vi "TSCAN_Periodic_Sending.vi"(10 "Data":T2={"Communication message"={"Sender"="", "receiver"="", "message"="", "data"=variant}, "Data"={"Config_parameter"={"Bus_Type"=0, "Channel"=1, "Channels used"=1, "DLL_PATH"=path "", "Read message type"=1, "REC_Channel"=0}, "Send_parameter"={"SendData"=[0, 0, 0, 0, 0, 0, 0, 0, 0, 0, 0, 0, 0, 0, 0, 0, 0, 0, 0, 0, 0, 0, 0, 0, 0, 0, 0, 0, 0, 0, 0, 0, 0, 0, 0, 0, 0, 0, 0, 0, 0, 0, 0, 0, 0, 0, 0, 0, 0, 0, 0, 0, 0, 0, 0, 0, 0, 0, 0, 0, 0, 0, 0, 0, 0, 0, 0, 0, 0, 0, 0, 0, 0, 0, 0], "Data Length"=15, "ID"=0, "Frame Format"=0, "Frame Type"=0, "BRS"=enum."Close", "FD Frame"=0, "async&sync"=enum."async", "Timeout"=0}, "DBC_Ctr"={"DBC Path"=path "", "DBC loading channel"=0, "DatabaseId"=0, "DBMessages"=[], "DBSignals"=[]}, "CAN_Config_Array"=[], "CANFD_Config_Array"=[], "CAN_Config_Regs_Array"=[], "CANFD_Config_Regs_Array"=[], "Blf_Log"={"Blf_Log_PATH"=path ""}, "UDS"={"UDS Control"={"UDS Channel Index"=0, "Request ID"=1992, "Response ID"=2015, "Request ID (Func)"=1, "Session Mode"=1, "Reset Mode"=255, "DTC Mask"=0, "GropOfDTC"=0, "Seed Level"=2, "Seed"=[], "Key Level"=0, "Key"=[], "Read Identifier"=0, "UDS Read Data"=[], "ASCII Data"="", "Write Identifier"=0, "UDS Wrtie Data"=[], "IO Control Identifier"=1, "UDS IOControl Data"=[], "IO Control Mode"=0, "UDS IOControl Read Data"=[], "Routine Control Identifier"=0, "UDS RoutineControl Data"=[], "UDS RoutineControl Read Data"=[], "Routine Control Mode"=1, "SupportFDCAN"=TRUE, "time config"={"p2_timeout"=0, "p2_extended"=0, "s3_servertime"=0, "s3_clienttime"=0}, "ServiceLayer"={"FilledByte"=0, "STMin"=10, "BlockSize"=10, "FCDelay"=10, "MaxLength"=4095}, "Request"=[], "Respond"=[]}, "DiagModuleIndex"=1984}}, "CAN_Buffer"=[], "CANFD_Buffer"=[], "error in"={"status"=FALSE, "code"=0, "source"=""}, "CAN_Period_Datas"=[], "CANFD_period_Datas"=[], "CAN_Filtering_Datas"=[], "CANFD_Filtering_Datas"=[], "AsynCall?"=FALSE} {"Data"."UDS"."UDS Control"."Respond" format="%.0x"; "Data"."UDS"."UDS Control"."Request" format="%.0x"; "Data"."UDS"."UDS Control"."ServiceLayer"."FilledByte" format="%.0x"; "Data"."UDS"."UDS Control"."GropOfDTC" format="%.0x"; "Data"."UDS"."UDS Control"."DTC Mask" format="%.0x"; "Data"."UDS"."UDS Control"."UDS RoutineControl Read Data" format="%.0x"; "Data"."UDS"."UDS Control"."UDS RoutineControl Data" format="%.0x"; "Data"."UDS"."UDS Control"."Routine Control Identifier" format="%.0x"; "Data"."UDS"."UDS Control"."UDS IOControl Read Data" format="%.0x"; "Data"."UDS"."UDS Control"."UDS IOControl Data" format="%.0x"; "Data"."UDS"."UDS Control"."IO Control Identifier" format="%.0x"; "Data"."UDS"."UDS Control"."UDS Wrtie Data" format="%.0x"; "Data"."UDS"."UDS Control"."UDS Read Data" format="%.0x"; "Data"."UDS"."UDS Control"."Write Identifier" format="%.0x"; "Data"."UDS"."UDS Control"."Read Identifier" format="%.0x"; "Data"."UDS"."UDS Control"."Key" format="%.0x"; "Data"."UDS"."UDS Control"."Seed" format="%.0x"; "Data"."UDS"."UDS Control"."Request ID (Func)" format="%.0x"; "Data"."UDS"."UDS Control"."Response ID" format="%.0x"; "Data"."UDS"."UDS Control"."Request ID" format="%.0x"; "Data"."UDS"."UDS Control"."Session Mode" items=["DefaultSession"=1, "ProgrammingSession"=2, "ExtendedDiagnosticSession"=3]; "Data"."UDS"."UDS Control"."Reset Mode" items=["HardReset"=1, "keyOffOnReset"=2, "SoftReset"=3]; "Data"."UDS"."UDS Control"."IO Control Mode" items=["ReturnControlToECU", "ResetToDefault", "FreezeCurrentState", "ShortTermAdjustment"]; "Data"."UDS"."UDS Control"."Routine Control Mode" items=["Start routine"=1, "Stop routine"=2, "Request routine results"=3]; "Data"."CAN_Config_Regs_Array"."CAN configuration"."AAppChannel" items=["CHN1", "CHN2", "CHN3", "CHN4", "CHN5", "CHN6", "CHN7", "CHN8", "CHN9", "CHN10", "CHN11", "CHN12", "CHN13", "CHN14", "CHN15", "CHN16", "CHN17", "CHN18", "CHN19", "CHN20", "CHN21", "CHN22", "CHN23", "CHN24", "CHN25", "CHN26", "CHN27", "CHN28", "CHN29", "CHN30", "CHN31", "CHN32"]; "Data"."CAN_Config_Regs_Array"."CAN configuration"."AHwChannel" items=["CHN1", "CHN2", "CHN3", "CHN4", "CHN5", "CHN6", "CHN7", "CHN8", "CHN9", "CHN10", "CHN11", "CHN12", "CHN13", "CHN14", "CHN15", "CHN16", "CHN17", "CHN18", "CHN19", "CHN20", "CHN21", "CHN22", "CHN23", "CHN24", "CHN25", "CHN26", "CHN27", "CHN28", "CHN29", "CHN30", "CHN31", "CHN32"]; "Data"."CAN_Config_Regs_Array"."CAN configuration"."HardwareType" items=["BUS_UNKNOWN_TYPE", "TS_TCP_DEVICE", "XL_USB_DEVICE", "TS_USB_DEVICE", "PEAK_USB_DEVICE", "KVASER_USB_DEVICE", "ZLG_USB_DEVICE", "ICS_USB_DEVICE", "TS_TC1005_DEVICE", "CANABLE_USB_DEVICE", "TS_WIRELESS_OBD", "TS_USB_DEVICE_EX", "IXXAT_USB_DEVICE", "TS_ETH_IF_DEVICE", "TS_USB_IF_DEVICE", "BUS_DEV_TYPE_COUNT"]; "Data"."CANFD_Config_Regs_Array"."CANFD Configuration"."Hardware Type" items=["BUS_UNKNOWN_TYPE", "TS_TCP_DEVICE", "XL_USB_DEVICE", "TS_USB_DEVICE", "PEAK_USB_DEVICE", "KVASER_USB_DEVICE", "ZLG_USB_DEVICE", "ICS_USB_DEVICE", "TS_TC1005_DEVICE", "CANABLE_USB_DEVICE", "TS_WIRELESS_OBD", "TS_USB_DEVICE_EX", "IXXAT_USB_DEVICE", "TS_ETH_IF_DEVICE", "TS_USB_IF_DEVICE", "BUS_DEV_TYPE_COUNT"]; "Data"."CANFD_Config_Regs_Array"."CANFD Configuration"."AHwChannel" items=["CHN1", "CHN2", "CHN3", "CHN4", "CHN5", "CHN6", "CHN7", "CHN8", "CHN9", "CHN10", "CHN11", "CHN12", "CHN13", "CHN14", "CHN15", "CHN16", "CHN17", "CHN18", "CHN19", "CHN20", "CHN21", "CHN22", "CHN23", "CHN24", "CHN25", "CHN26", "CHN27", "CHN28", "CHN29", "CHN30", "CHN31", "CHN32"]; "Data"."CANFD_Config_Regs_Array"."CANFD Configuration"."AAppChannel" items=["CHN1", "CHN2", "CHN3", "CHN4", "CHN5", "CHN6", "CHN7", "CHN8", "CHN9", "CHN10", "CHN11", "CHN12", "CHN13", "CHN14", "CHN15", "CHN16", "CHN17", "CHN18", "CHN19", "CHN20", "CHN21", "CHN22", "CHN23", "CHN24", "CHN25", "CHN26", "CHN27", "CHN28", "CHN29", "CHN30", "CHN31", "CHN32"]; "Data"."CANFD_Config_Regs_Array"."CANFD Configuration"."AControllerType" items=["lfdtCAN", "lfdtISOFDCAN", "lfdtNonISOFDFDCAN"]; "Data"."CANFD_Config_Regs_Array"."CANFD Configuration"."AControllerMode" items=["lfdmNormal", "lfdmACKOff", "lfdmRestricted"]; "Data"."CANFD_Config_Array"."Hardware Type" items=["BUS_UNKNOWN_TYPE", "TS_TCP_DEVICE", "XL_USB_DEVICE", "TS_USB_DEVICE", "PEAK_USB_DEVICE", "KVASER_USB_DEVICE", "ZLG_USB_DEVICE", "ICS_USB_DEVICE", "TS_TC1005_DEVICE", "CANABLE_USB_DEVICE", "TS_WIRELESS_OBD", "TS_USB_DEVICE_EX", "IXXAT_USB_DEVICE", "TS_ETH_IF_DEVICE", "TS_USB_IF_DEVICE", "BUS_DEV_TYPE_COUNT"]; "Data"."CANFD_Config_Array"."AHwChannel" items=["CHN1", "CHN2", "CHN3", "CHN4", "CHN5", "CHN6", "CHN7", "CHN8", "CHN9", "CHN10", "CHN11", "CHN12", "CHN13", "CHN14", "CHN15", "CHN16", "CHN17", "CHN18", "CHN19", "CHN20", "CHN21", "CHN22", "CHN23", "CHN24", "CHN25", "CHN26", "CHN27", "CHN28", "CHN29", "CHN30", "CHN31", "CHN32"]; "Data"."CANFD_Config_Array"."AAppChannel" items=["CHN1", "CHN2", "CHN3", "CHN4", "CHN5", "CHN6", "CHN7", "CHN8", "CHN9", "CHN10", "CHN11", "CHN12", "CHN13", "CHN14", "CHN15", "CHN16", "CHN17", "CHN18", "CHN19", "CHN20", "CHN21", "CHN22", "CHN23", "CHN24", "CHN25", "CHN26", "CHN27", "CHN28", "CHN29", "CHN30", "CHN31", "CHN32"]; "Data"."CANFD_Config_Array"."AControllerType" items=["lfdtCAN", "lfdtISOFDCAN", "lfdtNonISOFDFDCAN"]; "Data"."CANFD_Config_Array"."AControllerMode" items=["lfdmNormal", "lfdmACKOff", "lfdmRestricted"]; "Data"."CAN_Config_Array"."AAppChannel" items=["CHN1", "CHN2", "CHN3", "CHN4", "CHN5", "CHN6", "CHN7", "CHN8", "CHN9", "CHN10", "CHN11", "CHN12", "CHN13", "CHN14", "CHN15", "CHN16", "CHN17", "CHN18", "CHN19", "CHN20", "CHN21", "CHN22", "CHN23", "CHN24", "CHN25", "CHN26", "CHN27", "CHN28", "CHN29", "CHN30", "CHN31", "CHN32"]; "Data"."CAN_Config_Array"."AHwChannel" items=["CHN1", "CHN2", "CHN3", "CHN4", "CHN5", "CHN6", "CHN7", "CHN8", "CHN9", "CHN10", "CHN11", "CHN12", "CHN13", "CHN14", "CHN15", "CHN16", "CHN17", "CHN18", "CHN19", "CHN20", "CHN21", "CHN22", "CHN23", "CHN24", "CHN25", "CHN26", "CHN27", "CHN28", "CHN29", "CHN30", "CHN31", "CHN32"]; "Data"."CAN_Config_Array"."HardwareType" items=["BUS_UNKNOWN_TYPE", "TS_TCP_DEVICE", "XL_USB_DEVICE", "TS_USB_DEVICE", "PEAK_USB_DEVICE", "KVASER_USB_DEVICE", "ZLG_USB_DEVICE", "ICS_USB_DEVICE", "TS_TC1005_DEVICE", "CANABLE_USB_DEVICE", "TS_WIRELESS_OBD", "TS_USB_DEVICE_EX", "IXXAT_USB_DEVICE", "TS_ETH_IF_DEVICE", "TS_USB_IF_DEVICE", "BUS_DEV_TYPE_COUNT"]; "Data"."DBC_Ctr"."DBSignals"."SignalList"."Message_Type" items=["CAN", "CANFD", "J1939"]; "Data"."DBC_Ctr"."DBSignals"."SignalList"."Mux_Type" items=["Normal", "multiplexor", "multiplexed"]; "Data"."DBC_Ctr"."DBSignals"."SignalList"."Is_Motorola" items=["Intel", "Motorola"]; "Data"."DBC_Ctr"."DBSignals"."SignalList"."Value_Type" items=["unsigned int", "signed int", "float", "double"]; "Data"."DBC_Ctr"."DBSignals"."SignalList"."ID" format="%.0x"; "Data"."DBC_Ctr"."DBMessages"."BRS" items=["No BRS", "BRS"]; "Data"."DBC_Ctr"."DBMessages"."ID" format="%.0x"; "Data"."DBC_Ctr"."DBMessages"."Type" items=["cftStdCAN", "cftExtCAN", "cftJ1939", "cftStdCANFD", "cftExtCANFD"]; "Data"."DBC_Ctr"."DBC loading channel" items=["CHN1", "CHN2", "CHN3", "CHN4", "CHN5", "CHN6", "CHN7", "CHN8", "CHN9", "CHN10", "CHN11", "CHN12", "CHN13", "CHN14", "CHN15", "CHN16", "CHN17", "CHN18", "CHN19", "CHN20", "CHN21", "CHN22", "CHN23", "CHN24", "CHN25", "CHN26", "CHN27", "CHN28", "CHN29", "CHN30", "CHN31", "CHN32"]; "Data"."Send_parameter"."FD Frame" items=["Ordinary CAN Data", "FD CAN Data"]; "Data"."Send_parameter"."Frame Type" items=["Standard Frame", "Extended Frame"]; "Data"."Send_parameter"."Frame Format" items=["Standard Frame", "Extended Frame"]; "Data"."Send_parameter"."ID" format="%x"; "Data"."Send_parameter"."Data Length" items=["0", "1", "2", "3", "4", "5", "6", "7", "8", "12", "16", "20", "24", "32", "48", "64"]; "Data"."Send_parameter"."SendData" format="%x"; "Data"."Config_parameter"."REC_Channel" items=["CHN1", "CHN2", "CHN3", "CHN4", "CHN5", "CHN6", "CHN7", "CHN8", "CHN9", "CHN10", "CHN11", "CHN12", "CHN13", "CHN14", "CHN15", "CHN16", "CHN17", "CHN18", "CHN19", "CHN20", "CHN21", "CHN22", "CHN23", "CHN24", "CHN25", "CHN26", "CHN27", "CHN28", "CHN29", "CHN30", "CHN31", "CHN32"]; "Data"."Config_parameter"."Read message type" items=["Only read received messages", "Receive&send messages"]; "Data"."Config_parameter"."Channels used" items=["1 Channel"=1, "2 Channels"=2, "3 Channels"=3, "4 Channels"=4, "5 Channels"=5, "6 Channels"=6, "7 Channels"=7, "8 Channels"=8, "9 Channels"=9, "10 Channels"=10, "11 Channels"=11, "12 Channels"=12, "13 Channels"=13, "14 Channels"=14, "15 Channels"=15, "16 Channels"=16]; "Data"."Config_parameter"."Channel" items=["Disable", "Enable"]; "Data"."Config_parameter"."Bus_Type" items=["CAN", "CANFD"]}, 11 "Sender":string="Demo") -> (2 "Data 2":T2={"Communication message"={"Sender"="", "receiver"="", "message"="", "data"=variant}, "Data"={"Config_parameter"={"Bus_Type"=0, "Channel"=1, "Channels used"=1, "DLL_PATH"=path "", "Read message type"=1, "REC_Channel"=0}, "Send_parameter"={"SendData"=[0, 0, 0, 0, 0, 0, 0, 0, 0, 0, 0, 0, 0, 0, 0, 0, 0, 0, 0, 0, 0, 0, 0, 0, 0, 0, 0, 0, 0, 0, 0, 0, 0, 0, 0, 0, 0, 0, 0, 0, 0, 0, 0, 0, 0, 0, 0, 0, 0, 0, 0, 0, 0, 0, 0, 0, 0, 0, 0, 0, 0, 0, 0, 0, 0, 0, 0, 0, 0, 0, 0, 0, 0, 0, 0], "Data Length"=15, "ID"=0, "Frame Format"=0, "Frame Type"=0, "BRS"=enum."Close", "FD Frame"=0, "async&sync"=enum."async", "Timeout"=0}, "DBC_Ctr"={"DBC Path"=path "", "DBC loading channel"=0, "DatabaseId"=0, "DBMessages"=[], "DBSignals"=[]}, "CAN_Config_Array"=[], "CANFD_Config_Array"=[], "CAN_Config_Regs_Array"=[], "CANFD_Config_Regs_Array"=[], "Blf_Log"={"Blf_Log_PATH"=path ""}, "UDS"={"UDS Control"={"UDS Channel Index"=0, "Request ID"=1992, "Response ID"=2015, "Request ID (Func)"=1, "Session Mode"=1, "Reset Mode"=255, "DTC Mask"=0, "GropOfDTC"=0, "Seed Level"=2, "Seed"=[], "Key Level"=0, "Key"=[], "Read Identifier"=0, "UDS Read Data"=[], "ASCII Data"="", "Write Identifier"=0, "UDS Wrtie Data"=[], "IO Control Identifier"=1, "UDS IOControl Data"=[], "IO Control Mode"=0, "UDS IOControl Read Data"=[], "Routine Control Identifier"=0, "UDS RoutineControl Data"=[], "UDS RoutineControl Read Data"=[], "Routine Control Mode"=1, "SupportFDCAN"=TRUE, "time config"={"p2_timeout"=0, "p2_extended"=0, "s3_servertime"=0, "s3_clienttime"=0}, "ServiceLayer"={"FilledByte"=0, "STMin"=10, "BlockSize"=10, "FCDelay"=10, "MaxLength"=4095}, "Request"=[], "Respond"=[]}, "DiagModuleIndex"=1984}}, "CAN_Buffer"=[], "CANFD_Buffer"=[], "error in"={"status"=FALSE, "code"=0, "source"=""}, "CAN_Period_Datas"=[], "CANFD_period_Datas"=[], "CAN_Filtering_Datas"=[], "CANFD_Filtering_Datas"=[], "AsynCall?"=FALSE} {"Data"."UDS"."UDS Control"."Respond" format="%.0x"; "Data"."UDS"."UDS Control"."Request" format="%.0x"; "Data"."UDS"."UDS Control"."ServiceLayer"."FilledByte" format="%.0x"; "Data"."UDS"."UDS Control"."GropOfDTC" format="%.0x"; "Data"."UDS"."UDS Control"."DTC Mask" format="%.0x"; "Data"."UDS"."UDS Control"."UDS RoutineControl Read Data" format="%.0x"; "Data"."UDS"."UDS Control"."UDS RoutineControl Data" format="%.0x"; "Data"."UDS"."UDS Control"."Routine Control Identifier" format="%.0x"; "Data"."UDS"."UDS Control"."UDS IOControl Read Data" format="%.0x"; "Data"."UDS"."UDS Control"."UDS IOControl Data" format="%.0x"; "Data"."UDS"."UDS Control"."IO Control Identifier" format="%.0x"; "Data"."UDS"."UDS Control"."UDS Wrtie Data" format="%.0x"; "Data"."UDS"."UDS Control"."UDS Read Data" format="%.0x"; "Data"."UDS"."UDS Control"."Write Identifier" format="%.0x"; "Data"."UDS"."UDS Control"."Read Identifier" format="%.0x"; "Data"."UDS"."UDS Control"."Key" format="%.0x"; "Data"."UDS"."UDS Control"."Seed" format="%.0x"; "Data"."UDS"."UDS Control"."Request ID (Func)" format="%.0x"; "Data"."UDS"."UDS Control"."Response ID" format="%.0x"; "Data"."UDS"."UDS Control"."Request ID" format="%.0x"; "Data"."UDS"."UDS Control"."Session Mode" items=["DefaultSession"=1, "ProgrammingSession"=2, "ExtendedDiagnosticSession"=3]; "Data"."UDS"."UDS Control"."Reset Mode" items=["HardReset"=1, "keyOffOnReset"=2, "SoftReset"=3]; "Data"."UDS"."UDS Control"."IO Control Mode" items=["ReturnControlToECU", "ResetToDefault", "FreezeCurrentState", "ShortTermAdjustment"]; "Data"."UDS"."UDS Control"."Routine Control Mode" items=["Start routine"=1, "Stop routine"=2, "Request routine results"=3]; "Data"."CAN_Config_Regs_Array"."CAN configuration"."AAppChannel" items=["CHN1", "CHN2", "CHN3", "CHN4", "CHN5", "CHN6", "CHN7", "CHN8", "CHN9", "CHN10", "CHN11", "CHN12", "CHN13", "CHN14", "CHN15", "CHN16", "CHN17", "CHN18", "CHN19", "CHN20", "CHN21", "CHN22", "CHN23", "CHN24", "CHN25", "CHN26", "CHN27", "CHN28", "CHN29", "CHN30", "CHN31", "CHN32"]; "Data"."CAN_Config_Regs_Array"."CAN configuration"."AHwChannel" items=["CHN1", "CHN2", "CHN3", "CHN4", "CHN5", "CHN6", "CHN7", "CHN8", "CHN9", "CHN10", "CHN11", "CHN12", "CHN13", "CHN14", "CHN15", "CHN16", "CHN17", "CHN18", "CHN19", "CHN20", "CHN21", "CHN22", "CHN23", "CHN24", "CHN25", "CHN26", "CHN27", "CHN28", "CHN29", "CHN30", "CHN31", "CHN32"]; "Data"."CAN_Config_Regs_Array"."CAN configuration"."HardwareType" items=["BUS_UNKNOWN_TYPE", "TS_TCP_DEVICE", "XL_USB_DEVICE", "TS_USB_DEVICE", "PEAK_USB_DEVICE", "KVASER_USB_DEVICE", "ZLG_USB_DEVICE", "ICS_USB_DEVICE", "TS_TC1005_DEVICE", "CANABLE_USB_DEVICE", "TS_WIRELESS_OBD", "TS_USB_DEVICE_EX", "IXXAT_USB_DEVICE", "TS_ETH_IF_DEVICE", "TS_USB_IF_DEVICE", "BUS_DEV_TYPE_COUNT"]; "Data"."CANFD_Config_Regs_Array"."CANFD Configuration"."Hardware Type" items=["BUS_UNKNOWN_TYPE", "TS_TCP_DEVICE", "XL_USB_DEVICE", "TS_USB_DEVICE", "PEAK_USB_DEVICE", "KVASER_USB_DEVICE", "ZLG_USB_DEVICE", "ICS_USB_DEVICE", "TS_TC1005_DEVICE", "CANABLE_USB_DEVICE", "TS_WIRELESS_OBD", "TS_USB_DEVICE_EX", "IXXAT_USB_DEVICE", "TS_ETH_IF_DEVICE", "TS_USB_IF_DEVICE", "BUS_DEV_TYPE_COUNT"]; "Data"."CANFD_Config_Regs_Array"."CANFD Configuration"."AHwChannel" items=["CHN1", "CHN2", "CHN3", "CHN4", "CHN5", "CHN6", "CHN7", "CHN8", "CHN9", "CHN10", "CHN11", "CHN12", "CHN13", "CHN14", "CHN15", "CHN16", "CHN17", "CHN18", "CHN19", "CHN20", "CHN21", "CHN22", "CHN23", "CHN24", "CHN25", "CHN26", "CHN27", "CHN28", "CHN29", "CHN30", "CHN31", "CHN32"]; "Data"."CANFD_Config_Regs_Array"."CANFD Configuration"."AAppChannel" items=["CHN1", "CHN2", "CHN3", "CHN4", "CHN5", "CHN6", "CHN7", "CHN8", "CHN9", "CHN10", "CHN11", "CHN12", "CHN13", "CHN14", "CHN15", "CHN16", "CHN17", "CHN18", "CHN19", "CHN20", "CHN21", "CHN22", "CHN23", "CHN24", "CHN25", "CHN26", "CHN27", "CHN28", "CHN29", "CHN30", "CHN31", "CHN32"]; "Data"."CANFD_Config_Regs_Array"."CANFD Configuration"."AControllerType" items=["lfdtCAN", "lfdtISOFDCAN", "lfdtNonISOFDFDCAN"]; "Data"."CANFD_Config_Regs_Array"."CANFD Configuration"."AControllerMode" items=["lfdmNormal", "lfdmACKOff", "lfdmRestricted"]; "Data"."CANFD_Config_Array"."Hardware Type" items=["BUS_UNKNOWN_TYPE", "TS_TCP_DEVICE", "XL_USB_DEVICE", "TS_USB_DEVICE", "PEAK_USB_DEVICE", "KVASER_USB_DEVICE", "ZLG_USB_DEVICE", "ICS_USB_DEVICE", "TS_TC1005_DEVICE", "CANABLE_USB_DEVICE", "TS_WIRELESS_OBD", "TS_USB_DEVICE_EX", "IXXAT_USB_DEVICE", "TS_ETH_IF_DEVICE", "TS_USB_IF_DEVICE", "BUS_DEV_TYPE_COUNT"]; "Data"."CANFD_Config_Array"."AHwChannel" items=["CHN1", "CHN2", "CHN3", "CHN4", "CHN5", "CHN6", "CHN7", "CHN8", "CHN9", "CHN10", "CHN11", "CHN12", "CHN13", "CHN14", "CHN15", "CHN16", "CHN17", "CHN18", "CHN19", "CHN20", "CHN21", "CHN22", "CHN23", "CHN24", "CHN25", "CHN26", "CHN27", "CHN28", "CHN29", "CHN30", "CHN31", "CHN32"]; "Data"."CANFD_Config_Array"."AAppChannel" items=["CHN1", "CHN2", "CHN3", "CHN4", "CHN5", "CHN6", "CHN7", "CHN8", "CHN9", "CHN10", "CHN11", "CHN12", "CHN13", "CHN14", "CHN15", "CHN16", "CHN17", "CHN18", "CHN19", "CHN20", "CHN21", "CHN22", "CHN23", "CHN24", "CHN25", "CHN26", "CHN27", "CHN28", "CHN29", "CHN30", "CHN31", "CHN32"]; "Data"."CANFD_Config_Array"."AControllerType" items=["lfdtCAN", "lfdtISOFDCAN", "lfdtNonISOFDFDCAN"]; "Data"."CANFD_Config_Array"."AControllerMode" items=["lfdmNormal", "lfdmACKOff", "lfdmRestricted"]; "Data"."CAN_Config_Array"."AAppChannel" items=["CHN1", "CHN2", "CHN3", "CHN4", "CHN5", "CHN6", "CHN7", "CHN8", "CHN9", "CHN10", "CHN11", "CHN12", "CHN13", "CHN14", "CHN15", "CHN16", "CHN17", "CHN18", "CHN19", "CHN20", "CHN21", "CHN22", "CHN23", "CHN24", "CHN25", "CHN26", "CHN27", "CHN28", "CHN29", "CHN30", "CHN31", "CHN32"]; "Data"."CAN_Config_Array"."AHwChannel" items=["CHN1", "CHN2", "CHN3", "CHN4", "CHN5", "CHN6", "CHN7", "CHN8", "CHN9", "CHN10", "CHN11", "CHN12", "CHN13", "CHN14", "CHN15", "CHN16", "CHN17", "CHN18", "CHN19", "CHN20", "CHN21", "CHN22", "CHN23", "CHN24", "CHN25", "CHN26", "CHN27", "CHN28", "CHN29", "CHN30", "CHN31", "CHN32"]; "Data"."CAN_Config_Array"."HardwareType" items=["BUS_UNKNOWN_TYPE", "TS_TCP_DEVICE", "XL_USB_DEVICE", "TS_USB_DEVICE", "PEAK_USB_DEVICE", "KVASER_USB_DEVICE", "ZLG_USB_DEVICE", "ICS_USB_DEVICE", "TS_TC1005_DEVICE", "CANABLE_USB_DEVICE", "TS_WIRELESS_OBD", "TS_USB_DEVICE_EX", "IXXAT_USB_DEVICE", "TS_ETH_IF_DEVICE", "TS_USB_IF_DEVICE", "BUS_DEV_TYPE_COUNT"]; "Data"."DBC_Ctr"."DBSignals"."SignalList"."Message_Type" items=["CAN", "CANFD", "J1939"]; "Data"."DBC_Ctr"."DBSignals"."SignalList"."Mux_Type" items=["Normal", "multiplexor", "multiplexed"]; "Data"."DBC_Ctr"."DBSignals"."SignalList"."Is_Motorola" items=["Intel", "Motorola"]; "Data"."DBC_Ctr"."DBSignals"."SignalList"."Value_Type" items=["unsigned int", "signed int", "float", "double"]; "Data"."DBC_Ctr"."DBSignals"."SignalList"."ID" format="%.0x"; "Data"."DBC_Ctr"."DBMessages"."BRS" items=["No BRS", "BRS"]; "Data"."DBC_Ctr"."DBMessages"."ID" format="%.0x"; "Data"."DBC_Ctr"."DBMessages"."Type" items=["cftStdCAN", "cftExtCAN", "cftJ1939", "cftStdCANFD", "cftExtCANFD"]; "Data"."DBC_Ctr"."DBC loading channel" items=["CHN1", "CHN2", "CHN3", "CHN4", "CHN5", "CHN6", "CHN7", "CHN8", "CHN9", "CHN10", "CHN11", "CHN12", "CHN13", "CHN14", "CHN15", "CHN16", "CHN17", "CHN18", "CHN19", "CHN20", "CHN21", "CHN22", "CHN23", "CHN24", "CHN25", "CHN26", "CHN27", "CHN28", "CHN29", "CHN30", "CHN31", "CHN32"]; "Data"."Send_parameter"."FD Frame" items=["Ordinary CAN Data", "FD CAN Data"]; "Data"."Send_parameter"."Frame Type" items=["Standard Frame", "Extended Frame"]; "Data"."Send_parameter"."Frame Format" items=["Standard Frame", "Extended Frame"]; "Data"."Send_parameter"."ID" format="%x"; "Data"."Send_parameter"."Data Length" items=["0", "1", "2", "3", "4", "5", "6", "7", "8", "12", "16", "20", "24", "32", "48", "64"]; "Data"."Send_parameter"."SendData" format="%x"; "Data"."Config_parameter"."REC_Channel" items=["CHN1", "CHN2", "CHN3", "CHN4", "CHN5", "CHN6", "CHN7", "CHN8", "CHN9", "CHN10", "CHN11", "CHN12", "CHN13", "CHN14", "CHN15", "CHN16", "CHN17", "CHN18", "CHN19", "CHN20", "CHN21", "CHN22", "CHN23", "CHN24", "CHN25", "CHN26", "CHN27", "CHN28", "CHN29", "CHN30", "CHN31", "CHN32"]; "Data"."Config_parameter"."Read message type" items=["Only read received messages", "Receive&send messages"]; "Data"."Config_parameter"."Channels used" items=["1 Channel"=1, "2 Channels"=2, "3 Channels"=3, "4 Channels"=4, "5 Channels"=5, "6 Channels"=6, "7 Channels"=7, "8 Channels"=8, "9 Channels"=9, "10 Channels"=10, "11 Channels"=11, "12 Channels"=12, "13 Channels"=13, "14 Channels"=14, "15 Channels"=15, "16 Channels"=16]; "Data"."Config_parameter"."Channel" items=["Disable", "Enable"]; "Data"."Config_parameter"."Bus_Type" items=["CAN", "CANFD"]})   [LabVIEW 2014]
uses:
  <vilib>/Utility/miscctls.llb/LVPointTypeDef.ctl
  Typedef/TSCAN_Config_parameter.ctl
  Typedef/TSCAN_Send_parameter.ctl
  Typedef/TSCAN_DBC_Ctr.ctl
  Utilities/Typedef/Hardware_Subtype.ctl
  Typedef/TSCAN_CAN_Configuration.ctl
  Typedef/TSCAN_CANFD_Configuration.ctl
  Typedef/TSCAN_CAN_CANFD_Demo_Data.ctl
  Typedef/TSCAN_CAN_CANFD_Demo_Data1.ctl
  Typedef/TLibCANFD.ctl
  Typedef/TLibCAN.ctl
  Typedef/TSCAN_CANFD_Configuration_Regs.ctl
  Typedef/TSCAN_CAN_Configuration_Regs.ctl
  All_Control/Typedef/Hardware Type.ctl
  All_Control/Typedef/Blf_Log.ctl
  DataBase/Typedef/DBSignal.ctl
  DataBase/Typedef/DBMessage.ctl
  Diagnosis/Typedef/UDS Control.ctl
  Diagnosis/Typedef/UDS Cluster.ctl
panel:
  in  "Channel":i32(ring) items=["CHN1", "CHN2", "CHN3", "CHN4", "CHN5", "CHN6", "CHN7", "CHN8", "CHN9", "CHN10", "CHN11", "CHN12", "CHN13", "CHN14", "CHN15", "CHN16", "CHN17", "CHN18", "CHN19", "CHN20", "CHN21", "CHN22", "CHN23", "CHN24", "CHN25", "CHN26", "CHN27", "CHN28", "CHN29", "CHN30", "CHN31", "CHN32"]
  out "CAN_Period_Datas":T1(array[cluster])
  in  "APeriodMS":dbl
  in  "BRS":enum16{"Close", "Open"}(ring)
  in  "FD Frame":u8(ring) items=["Ordinary CAN Data", "FD CAN Data"]
  in  "Frame Type":u8(ring) items=["Data Frame", "Remote Frame", ""]
  in  "Frame Format":u8(ring) items=["Standard Frame", "Extended Frame"]
  in  "ID":i32 format="%x"
  in  "Data Length":i32(ring)=15 items=["0", "1", "2", "3", "4", "5", "6", "7", "8", "12", "16", "20", "24", "32", "48", "64"]
  in  "SendData":u8[](array[numeric])=[0, 0, 0, 0, 0, 0, 0, 0, 0, 0, 0, 0, 0, 0, 0, 0, 0, 0, 0, 0, 0, 0, 0, 0, 0, 0, 0, 0, 0, 0, 0, 0, 0, 0, 0, 0, 0, 0, 0, 0, 0, 0, 0, 0, 0, 0, 0, 0, 0, 0, 0, 0, 0, 0, 0, 0, 0, 0, 0, 0, 0, 0, 0, 0, 0, 0, 0, 0, 0, 0, 0, 0, 0, 0, 0] format="%x"
  in  "Data_Display":i32(listbox)=-1
  in  "Remove":bool
  in  "Add":bool
  in  "STOP":bool
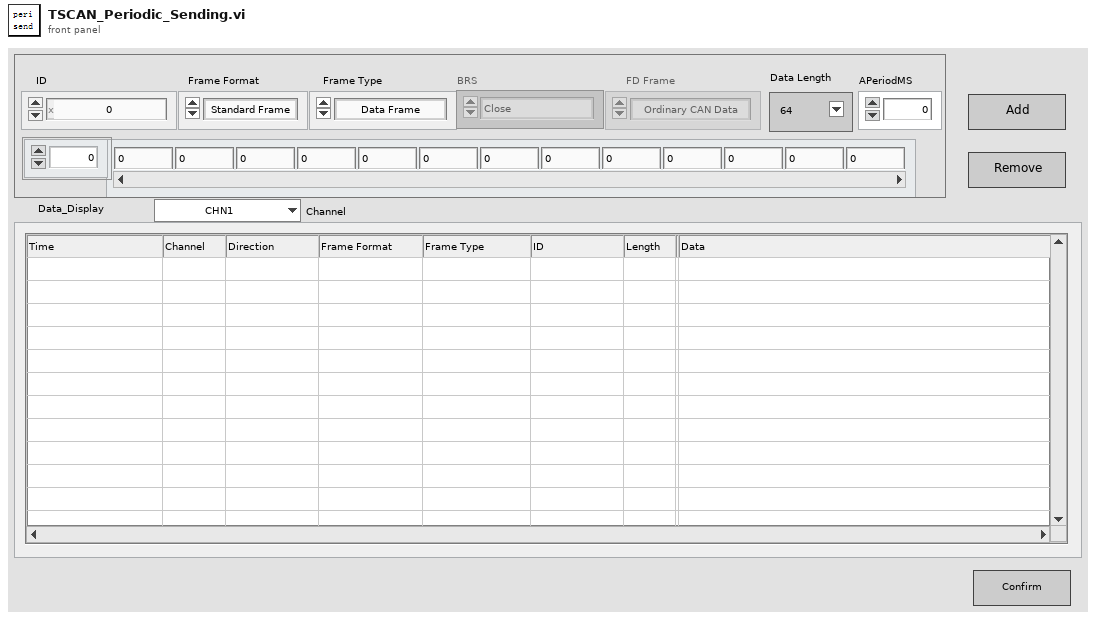
[diagram p1: front panel]
types:
  T1 = cluster{"FIdxChn":u8, "FProperties":u8, "FDLC":u8, "FReserved":u8, "FIdentifier":i32, "FTimeUS":u64, "FData":cluster{"Data0":u8, "Data1":u8, "Data2":u8, "Data3":u8, "Data4":u8, "Data5":u8, "Data6":u8, "Data7":u8}}[]
  T2 = typedef "TSCAN_CAN_CANFD_Demo_Data1.ctl" = cluster{"Communication message":cluster{"Sender":string, "receiver":string, "message":string, "data":variant}, "Data":T3, "CAN_Buffer":cluster{"FIdxChn":u8, "FProperties":u8, "FDLC":u8, "FReserved":u8, "FIdentifier":i32, "FTimeUS":u64, "FData":cluster{"Data0":u8, "Data1":u8, "Data2":u8, "Data3":u8, "Data4":u8, "Data5":u8, "Data6":u8, "Data7":u8}}[], "CANFD_Buffer":cluster{"FIdxChn":u8, "FProperties":u8, "FDLC":u8, "FReserved":u8, "FIdentifier":i32, "FTimeUS":u64, "FDatas":cluster{"Initialize array[0]":u8, "Initialize array[1]":u8, "Initialize array[2]":u8, "Initialize array[3]":u8, "Initialize array[4]":u8, "Initialize array[5]":u8, "Initialize array[6]":u8, "Initialize array[7]":u8, "Initialize array[8]":u8, "Initialize array[9]":u8, "Initialize array[10]":u8, "Initialize array[11]":u8, "Initialize array[12]":u8, "Initialize array[13]":u8, "Initialize array[14]":u8, "Initialize array[15]":u8, "Initialize array[16]":u8, "Initialize array[17]":u8, "Initialize array[18]":u8, "Initialize array[19]":u8, "Initialize array[20]":u8, "Initialize array[21]":u8, "Initialize array[22]":u8, "Initialize array[23]":u8, "Initialize array[24]":u8, "Initialize array[25]":u8, "Initialize array[26]":u8, "Initialize array[27]":u8, "Initialize array[28]":u8, "Initialize array[29]":u8, "Initialize array[30]":u8, "Initialize array[31]":u8, "Initialize array[32]":u8, "Initialize array[33]":u8, "Initialize array[34]":u8, "Initialize array[35]":u8, "Initialize array[36]":u8, "Initialize array[37]":u8, "Initialize array[38]":u8, "Initialize array[39]":u8, "Initialize array[40]":u8, "Initialize array[41]":u8, "Initialize array[42]":u8, "Initialize array[43]":u8, "Initialize array[44]":u8, "Initialize array[45]":u8, "Initialize array[46]":u8, "Initialize array[47]":u8, "Initialize array[48]":u8, "Initialize array[49]":u8, "Initialize array[50]":u8, "Initialize array[51]":u8, "Initialize array[52]":u8, "Initialize array[53]":u8, "Initialize array[54]":u8, "Initialize array[55]":u8, "Initialize array[56]":u8, "Initialize array[57]":u8, "Initialize array[58]":u8, "Initialize array[59]":u8, "Initialize array[60]":u8, "Initialize array[61]":u8, "Initialize array[62]":u8, "Initialize array[63]":u8}}[], "error in":errorcluster, "CAN_Period_Datas":cluster{"FIdxChn":u8, "FProperties":u8, "FDLC":u8, "FReserved":u8, "FIdentifier":i32, "FTimeUS":u64, "FData":cluster{"Data0":u8, "Data1":u8, "Data2":u8, "Data3":u8, "Data4":u8, "Data5":u8, "Data6":u8, "Data7":u8}}[], "CANFD_period_Datas":cluster{"FIdxChn":u8, "FProperties":u8, "FDLC":u8, "FReserved":u8, "FIdentifier":i32, "FTimeUS":u64, "FDatas":cluster{"Initialize array[0]":u8, "Initialize array[1]":u8, "Initialize array[2]":u8, "Initialize array[3]":u8, "Initialize array[4]":u8, "Initialize array[5]":u8, "Initialize array[6]":u8, "Initialize array[7]":u8, "Initialize array[8]":u8, "Initialize array[9]":u8, "Initialize array[10]":u8, "Initialize array[11]":u8, "Initialize array[12]":u8, "Initialize array[13]":u8, "Initialize array[14]":u8, "Initialize array[15]":u8, "Initialize array[16]":u8, "Initialize array[17]":u8, "Initialize array[18]":u8, "Initialize array[19]":u8, "Initialize array[20]":u8, "Initialize array[21]":u8, "Initialize array[22]":u8, "Initialize array[23]":u8, "Initialize array[24]":u8, "Initialize array[25]":u8, "Initialize array[26]":u8, "Initialize array[27]":u8, "Initialize array[28]":u8, "Initialize array[29]":u8, "Initialize array[30]":u8, "Initialize array[31]":u8, "Initialize array[32]":u8, "Initialize array[33]":u8, "Initialize array[34]":u8, "Initialize array[35]":u8, "Initialize array[36]":u8, "Initialize array[37]":u8, "Initialize array[38]":u8, "Initialize array[39]":u8, "Initialize array[40]":u8, "Initialize array[41]":u8, "Initialize array[42]":u8, "Initialize array[43]":u8, "Initialize array[44]":u8, "Initialize array[45]":u8, "Initialize array[46]":u8, "Initialize array[47]":u8, "Initialize array[48]":u8, "Initialize array[49]":u8, "Initialize array[50]":u8, "Initialize array[51]":u8, "Initialize array[52]":u8, "Initialize array[53]":u8, "Initialize array[54]":u8, "Initialize array[55]":u8, "Initialize array[56]":u8, "Initialize array[57]":u8, "Initialize array[58]":u8, "Initialize array[59]":u8, "Initialize array[60]":u8, "Initialize array[61]":u8, "Initialize array[62]":u8, "Initialize array[63]":u8}}[], "CAN_Filtering_Datas":cluster{"FIdxChn":u8, "FProperties":u8, "FDLC":u8, "FReserved":u8, "FIdentifier":i32, "FTimeUS":u64, "FData":cluster{"Data0":u8, "Data1":u8, "Data2":u8, "Data3":u8, "Data4":u8, "Data5":u8, "Data6":u8, "Data7":u8}}[], "CANFD_Filtering_Datas":cluster{"FIdxChn":u8, "FProperties":u8, "FDLC":u8, "FReserved":u8, "FIdentifier":i32, "FTimeUS":u64, "FDatas":cluster{"Initialize array[0]":u8, "Initialize array[1]":u8, "Initialize array[2]":u8, "Initialize array[3]":u8, "Initialize array[4]":u8, "Initialize array[5]":u8, "Initialize array[6]":u8, "Initialize array[7]":u8, "Initialize array[8]":u8, "Initialize array[9]":u8, "Initialize array[10]":u8, "Initialize array[11]":u8, "Initialize array[12]":u8, "Initialize array[13]":u8, "Initialize array[14]":u8, "Initialize array[15]":u8, "Initialize array[16]":u8, "Initialize array[17]":u8, "Initialize array[18]":u8, "Initialize array[19]":u8, "Initialize array[20]":u8, "Initialize array[21]":u8, "Initialize array[22]":u8, "Initialize array[23]":u8, "Initialize array[24]":u8, "Initialize array[25]":u8, "Initialize array[26]":u8, "Initialize array[27]":u8, "Initialize array[28]":u8, "Initialize array[29]":u8, "Initialize array[30]":u8, "Initialize array[31]":u8, "Initialize array[32]":u8, "Initialize array[33]":u8, "Initialize array[34]":u8, "Initialize array[35]":u8, "Initialize array[36]":u8, "Initialize array[37]":u8, "Initialize array[38]":u8, "Initialize array[39]":u8, "Initialize array[40]":u8, "Initialize array[41]":u8, "Initialize array[42]":u8, "Initialize array[43]":u8, "Initialize array[44]":u8, "Initialize array[45]":u8, "Initialize array[46]":u8, "Initialize array[47]":u8, "Initialize array[48]":u8, "Initialize array[49]":u8, "Initialize array[50]":u8, "Initialize array[51]":u8, "Initialize array[52]":u8, "Initialize array[53]":u8, "Initialize array[54]":u8, "Initialize array[55]":u8, "Initialize array[56]":u8, "Initialize array[57]":u8, "Initialize array[58]":u8, "Initialize array[59]":u8, "Initialize array[60]":u8, "Initialize array[61]":u8, "Initialize array[62]":u8, "Initialize array[63]":u8}}[], "AsynCall?":bool}
  T3 = typedef "TSCAN_CAN_CANFD_Demo_Data.ctl" = cluster{"Config_parameter":T4, "Send_parameter":T5, "DBC_Ctr":T6, "CAN_Config_Array":T9[], "CANFD_Config_Array":T12[], "CAN_Config_Regs_Array":T13[], "CANFD_Config_Regs_Array":T14[], "Blf_Log":T15, "UDS":T16}
  T4 = typedef "TSCAN_Config_parameter.ctl" = cluster{"Bus_Type":u16, "Channel":i32, "Channels used":u16, "DLL_PATH":path, "Read message type":u16, "REC_Channel":i32}
  T5 = typedef "TSCAN_Send_parameter.ctl" = cluster{"SendData":u8[], "Data Length":i32, "ID":i32, "Frame Format":u8, "Frame Type":u8, "BRS":enum16{"Close", "Open"}, "FD Frame":u8, "async&sync":enum16{"async", "sync"}, "Timeout":u16}
  T6 = typedef "TSCAN_DBC_Ctr.ctl" = cluster{"DBC Path":path, "DBC loading channel":i32, "DatabaseId":u32, "DBMessages":T7[], "DBSignals":cluster{"MessageName":string, "SignalList":T8[]}[]}
  T7 = typedef "DBMessage.ctl" = cluster{"Type":u16, "DLC":i32, "ID":i32, "CycleTime":dbl, "Name":string, "Comment":string, "TX_Node_Index":i32, "Owned_Signal_List_Count ":i32, "Owned_Signal_List_Signal_Index":i32, "BRS":i32}
  T8 = typedef "DBSignal.ctl" = cluster{"ID":i32, "Value_Type":i32, "Is_Motorola":i32, "ValTab_Index":i32, "Mux_Type":i32, "Mux_Value":dbl, "Layout_Start":i32, "Length":i32, "Factor":dbl, "Offset":dbl, "InitValue":dbl, "Min":dbl, "Max":dbl, "Name":string, "Unit":string, "Comment":string, "Message_Index":i32, "Message_Type":i32}
  T9 = typedef "TSCAN_CAN_Configuration.ctl" = cluster{"HardwareType":T10, "Hardware Subtype":T11, "ABaudrateKbps":sgl, "AListenOnly":enum16{"Normal", "ListenOnly"}, "Int120Ohm":enum16{"Disable", "Enable"}, "EnableChannel":enum16{"Disable", "Enable"}, "AHwChannel":i32, "AAppChannel":i32, "AldHW":i32}
  T10 = typedef "Hardware Type.ctl" = i32
  T11 = typedef "Hardware_Subtype.ctl" = enum16{"TS_UNKNOWN_DEVICE", "TSCAN_PRO", "TSCAN_Lite1", "TC1001", "TL1001", "TC1011", "TM5011", "TC1002", "TC1014", "TSCANFD2517", "TC1026", "TC1016", "TC1012", "TC1013", "TLog1002", "TC1034", "TC1018", "GW2116", "TC2115", "MP1013", "TC1113", "TC1114", "TP1013", "TC1017", "TP1018", "TF10XX", "TL1004_FD_4_LIN_2", "TE1051", "TP1051", "TP1034", "TTS9015", "TP1026", "TTS1026", "TTS1034", "TTS1018", "TL1011", "TTS1015_LiAuto", "TTS1013_LiAuto", "TTS1016Pro", "TC1054Pro", "TC1054", "TLog1038", "TO1013", "TC1034Pro", "TC1018Pro", "TC1038Pro", "TS_DEV_END"}
  T12 = typedef "TSCAN_CANFD_Configuration.ctl" = cluster{"Hardware Type":T10, "Hardware Subtype":T11, "AArbRateKbps":sgl, "AListenOnly":enum16{"Normal", "ListenOnly"}, "Int120Ohm":enum16{"Disable", "Enable"}, "EnableChannel":enum16{"Disable", "Enable"}, "AHwChannel":i32, "AAppChannel":i32, "ADataRateKbps":sgl, "AControllerType":i32, "AControllerMode":i32, "AldHW":i32}
  T13 = typedef "TSCAN_CAN_Configuration_Regs.ctl" = cluster{"CAN_Sampling point":cluster{"ASEG1":i32, "ASEG2":i32, "APrescaler":i32, "ASJW":i32}, "CAN configuration":T9}
  T14 = typedef "TSCAN_CANFD_Configuration_Regs.ctl" = cluster{"CANFD Configuration":T12, "CANFD_Sampling point":cluster{"AArbSEG1":i32, "AArbSEG2":i32, "AArbPrescaler":i32, "AArbSJW":i32, "ADataSEG1":i32, "ADataSEG2":i32, "ADataPrescaler":i32, "ADataSJW":i32}}
  T15 = typedef "Blf_Log.ctl" = cluster{"Blf_Log_PATH":path}
  T16 = typedef "UDS Cluster.ctl" = cluster{"UDS Control":T17, "DiagModuleIndex":i32}
  T17 = typedef "UDS Control.ctl" = cluster{"UDS Channel Index":u32, "Request ID":u32, "Response ID":u32, "Request ID (Func)":u32, "Session Mode":u8, "Reset Mode":u8, "DTC Mask":u8, "GropOfDTC":u32, "Seed Level":i32, "Seed":u8[], "Key Level":i32, "Key":u8[], "Read Identifier":u16, "UDS Read Data":u8[], "ASCII Data":string, "Write Identifier":u16, "UDS Wrtie Data":u8[], "IO Control Identifier":u16, "UDS IOControl Data":u8[], "IO Control Mode":u8, "UDS IOControl Read Data":u8[], "Routine Control Identifier":u16, "UDS RoutineControl Data":u8[], "UDS RoutineControl Read Data":u8[], "Routine Control Mode":u8, "SupportFDCAN":bool, "time config":cluster{"p2_timeout":i32, "p2_extended":i32, "s3_servertime":i32, "s3_clienttime":i32}, "ServiceLayer":cluster{"FilledByte":u8, "STMin":i32, "BlockSize":i32, "FCDelay":i32, "MaxLength":i32}, "Request":u8[], "Respond":u8[]}
  T18 = cluster{"Sender":string, "receiver":string, "message":string, "data":variant}
  T19 = typedef "LVPointTypeDef.ctl" = cluster{"Horizontal":i16, "Vertical":i16}
  T20 = enum8{"Enabled", "Disabled", "Disabled and Grayed Out"}
  T21 = cluster{"FIdxChn":u8, "FProperties":u8, "FDLC":u8, "FReserved":u8, "FIdentifier":i32, "FTimeUS":u64, "FDatas":cluster{"Initialize array[0]":u8, "Initialize array[1]":u8, "Initialize array[2]":u8, "Initialize array[3]":u8, "Initialize array[4]":u8, "Initialize array[5]":u8, "Initialize array[6]":u8, "Initialize array[7]":u8, "Initialize array[8]":u8, "Initialize array[9]":u8, "Initialize array[10]":u8, "Initialize array[11]":u8, "Initialize array[12]":u8, "Initialize array[13]":u8, "Initialize array[14]":u8, "Initialize array[15]":u8, "Initialize array[16]":u8, "Initialize array[17]":u8, "Initialize array[18]":u8, "Initialize array[19]":u8, "Initialize array[20]":u8, "Initialize array[21]":u8, "Initialize array[22]":u8, "Initialize array[23]":u8, "Initialize array[24]":u8, "Initialize array[25]":u8, "Initialize array[26]":u8, "Initialize array[27]":u8, "Initialize array[28]":u8, "Initialize array[29]":u8, "Initialize array[30]":u8, "Initialize array[31]":u8, "Initialize array[32]":u8, "Initialize array[33]":u8, "Initialize array[34]":u8, "Initialize array[35]":u8, "Initialize array[36]":u8, "Initialize array[37]":u8, "Initialize array[38]":u8, "Initialize array[39]":u8, "Initialize array[40]":u8, "Initialize array[41]":u8, "Initialize array[42]":u8, "Initialize array[43]":u8, "Initialize array[44]":u8, "Initialize array[45]":u8, "Initialize array[46]":u8, "Initialize array[47]":u8, "Initialize array[48]":u8, "Initialize array[49]":u8, "Initialize array[50]":u8, "Initialize array[51]":u8, "Initialize array[52]":u8, "Initialize array[53]":u8, "Initialize array[54]":u8, "Initialize array[55]":u8, "Initialize array[56]":u8, "Initialize array[57]":u8, "Initialize array[58]":u8, "Initialize array[59]":u8, "Initialize array[60]":u8, "Initialize array[61]":u8, "Initialize array[62]":u8, "Initialize array[63]":u8}}[]
  T22 = typedef "TLibCAN.ctl" = cluster{"AIdxchn":u8, "AId":i32, "AIsStd":u8, "AIsData":u8, "ADLC":u8, "ADataArray":cluster{"Data0":u8, "Data1":u8, "Data2":u8, "Data3":u8, "Data4":u8, "Data5":u8, "Data6":u8, "Data7":u8}}
  T23 = typedef "TLibCANFD.ctl" = cluster{"AIdxchn":u8, "AId":i32, "AIsStd":u8, "BRS":enum16{"Close", "Open"}, "AIsData":u8, "ADLC":i32, "AIsFD":enum16{"Classic CAN Message", "FD CAN Message"}, "FDatas":cluster{"Initialize array[0]":u8, "Initialize array[1]":u8, "Initialize array[2]":u8, "Initialize array[3]":u8, "Initialize array[4]":u8, "Initialize array[5]":u8, "Initialize array[6]":u8, "Initialize array[7]":u8, "Initialize array[8]":u8, "Initialize array[9]":u8, "Initialize array[10]":u8, "Initialize array[11]":u8, "Initialize array[12]":u8, "Initialize array[13]":u8, "Initialize array[14]":u8, "Initialize array[15]":u8, "Initialize array[16]":u8, "Initialize array[17]":u8, "Initialize array[18]":u8, "Initialize array[19]":u8, "Initialize array[20]":u8, "Initialize array[21]":u8, "Initialize array[22]":u8, "Initialize array[23]":u8, "Initialize array[24]":u8, "Initialize array[25]":u8, "Initialize array[26]":u8, "Initialize array[27]":u8, "Initialize array[28]":u8, "Initialize array[29]":u8, "Initialize array[30]":u8, "Initialize array[31]":u8, "Initialize array[32]":u8, "Initialize array[33]":u8, "Initialize array[34]":u8, "Initialize array[35]":u8, "Initialize array[36]":u8, "Initialize array[37]":u8, "Initialize array[38]":u8, "Initialize array[39]":u8, "Initialize array[40]":u8, "Initialize array[41]":u8, "Initialize array[42]":u8, "Initialize array[43]":u8, "Initialize array[44]":u8, "Initialize array[45]":u8, "Initialize array[46]":u8, "Initialize array[47]":u8, "Initialize array[48]":u8, "Initialize array[49]":u8, "Initialize array[50]":u8, "Initialize array[51]":u8, "Initialize array[52]":u8, "Initialize array[53]":u8, "Initialize array[54]":u8, "Initialize array[55]":u8, "Initialize array[56]":u8, "Initialize array[57]":u8, "Initialize array[58]":u8, "Initialize array[59]":u8, "Initialize array[60]":u8, "Initialize array[61]":u8, "Initialize array[62]":u8, "Initialize array[63]":u8}}
  T24 = cluster{"SendData[0]":u8, "SendData[1]":u8, "SendData[2]":u8, "SendData[3]":u8, "SendData[4]":u8, "SendData[5]":u8, "SendData[6]":u8, "SendData[7]":u8}
  T25 = cluster{"SendData[0]":u8, "SendData[1]":u8, "SendData[2]":u8, "SendData[3]":u8, "SendData[4]":u8, "SendData[5]":u8, "SendData[6]":u8, "SendData[7]":u8, "SendData[8]":u8, "SendData[9]":u8, "SendData[10]":u8, "SendData[11]":u8, "SendData[12]":u8, "SendData[13]":u8, "SendData[14]":u8, "SendData[15]":u8, "SendData[16]":u8, "SendData[17]":u8, "SendData[18]":u8, "SendData[19]":u8, "SendData[20]":u8, "SendData[21]":u8, "SendData[22]":u8, "SendData[23]":u8, "SendData[24]":u8, "SendData[25]":u8, "SendData[26]":u8, "SendData[27]":u8, "SendData[28]":u8, "SendData[29]":u8, "SendData[30]":u8, "SendData[31]":u8, "SendData[32]":u8, "SendData[33]":u8, "SendData[34]":u8, "SendData[35]":u8, "SendData[36]":u8, "SendData[37]":u8, "SendData[38]":u8, "SendData[39]":u8, "SendData[40]":u8, "SendData[41]":u8, "SendData[42]":u8, "SendData[43]":u8, "SendData[44]":u8, "SendData[45]":u8, "SendData[46]":u8, "SendData[47]":u8, "SendData[48]":u8, "SendData[49]":u8, "SendData[50]":u8, "SendData[51]":u8, "SendData[52]":u8, "SendData[53]":u8, "SendData[54]":u8, "SendData[55]":u8, "SendData[56]":u8, "SendData[57]":u8, "SendData[58]":u8, "SendData[59]":u8, "SendData[60]":u8, "SendData[61]":u8, "SendData[62]":u8, "SendData[63]":u8}
  T26 = enum32{"invalid app kind", "Development System", "Run Time System", "Student Edition", "Embedded LabVIEW", "Evaluation", "Custom"}
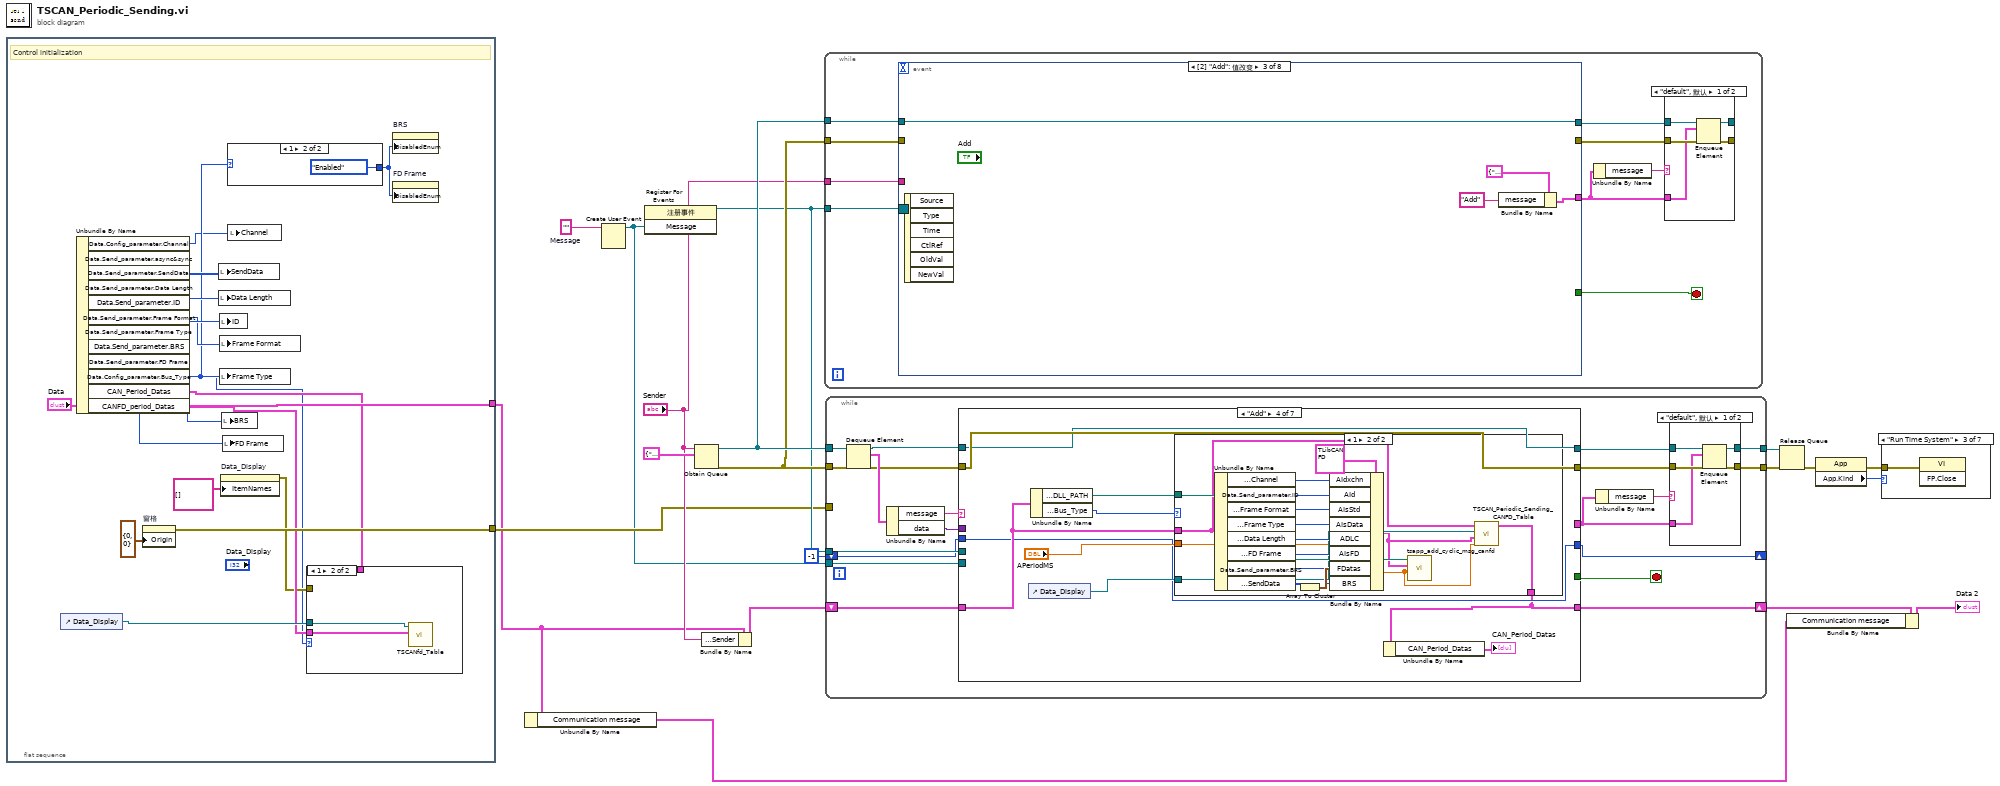
[diagram p0: block diagram]
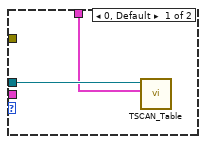
[diagram p2: hidden frame]
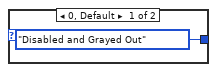
[diagram p3: hidden frame]
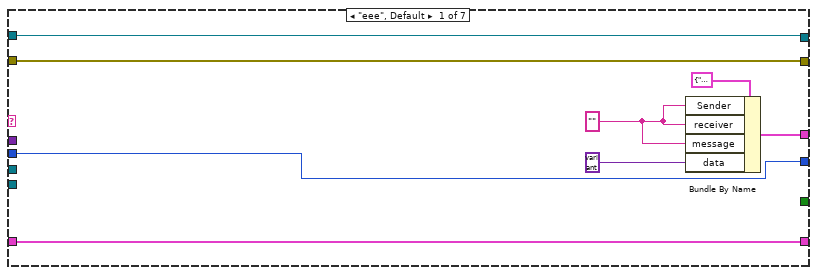
[diagram p11: hidden frame]
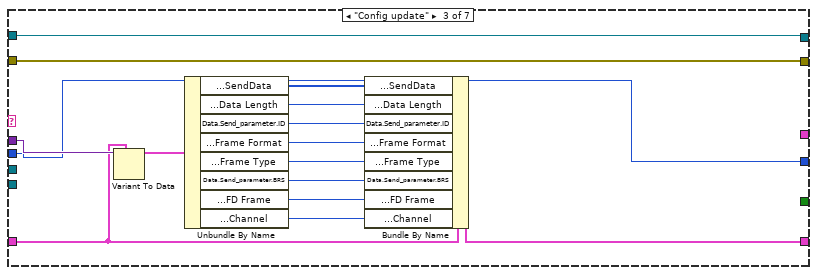
[diagram p13: hidden frame]
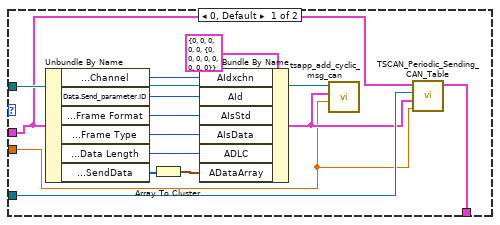
[diagram p14: hidden frame]
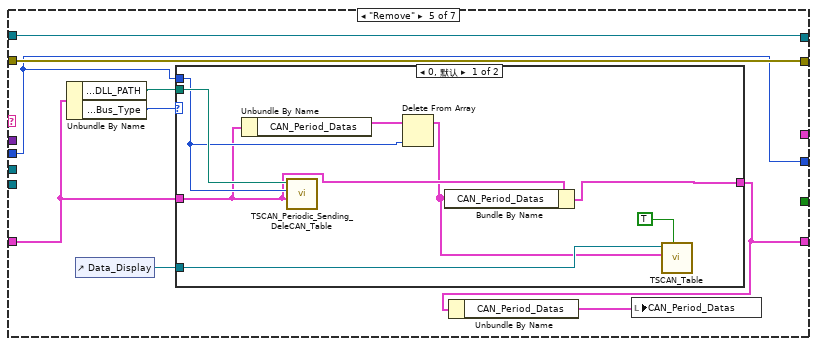
[diagram p15: hidden frame]
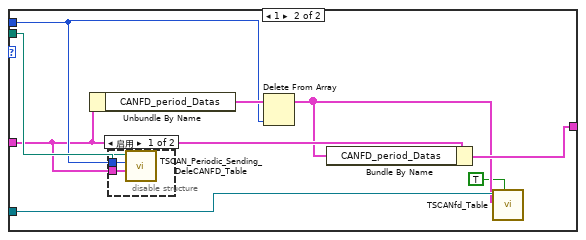
[diagram p16: hidden frame]
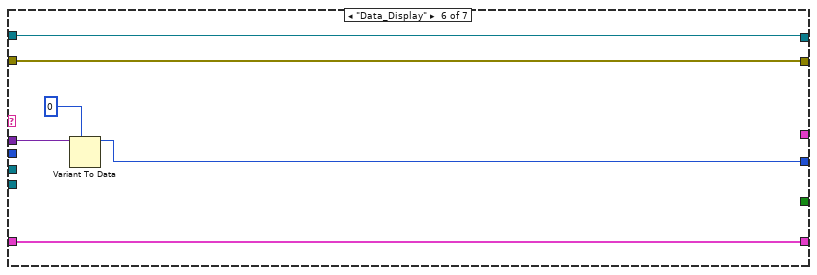
[diagram p18: hidden frame]
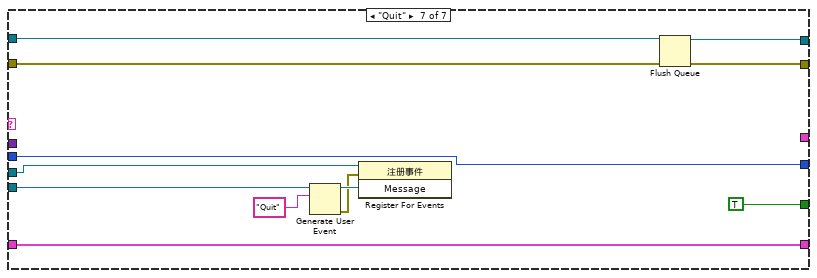
[diagram p19: hidden frame]
diagram:
  w9 = ""  # Message
  n1 = flat-sequence {
    tunnel: [w36] -> w7
    tunnel: ["Data"] -> w3
    frame #0 {
      # "Control initialization"
      n2 = control-ref of="Data_Display"() -> ()  [unwired: 1 out]
      n3 = control-ref of="Data_Display"() -> (w25:refnum<vi>)
      n4 = Unbundle By Name("Data") -> ("Data.Config_parameter.Channel"=w20:i32, "Data.Send_parameter.SendData"=w34:u8[], "Data.Send_parameter.Data Length"=w33:i32, "Data.Send_parameter.ID"=w32:i32, "Data.Send_parameter.Frame Format"=w31:u8, "Data.Send_parameter.Frame Type"=w30:u8, "Data.Send_parameter.BRS"=w29:enum16{"Close", "Open"}, "Data.Send_parameter.FD Frame"=w26:u8, "Data.Config_parameter.Bus_Type"=w21:u16, "CAN_Period_Datas"=w24:T1, "CANFD_period_Datas"=w23:T21)  [unwired: 1 out]
      n5 = property on="窗格" class="Pane"("Origin"=T19 {"Horizontal"=0, "Vertical"=0} ("原点")) -> (error out=w36:errorcluster)  [unwired: 2 in, 1 out]
      n6 = local write "SendData"(w34) -> ()
      n7 = local write "Data Length"(w33) -> ()
      n8 = local write "ID"(w32) -> ()
      n9 = local write "Frame Format"(w31) -> ()
      n10 = local write "Frame Type"(w30) -> ()
      n11 = property on="Data_Display" class="MCListbox (严格)"("ItemNames"=string[][] [] ("项名")) -> (error out=w22:errorcluster)  [unwired: 2 in, 1 out]
      n12 = local write "BRS"(w29) -> ()
      n13 = local write "FD Frame"(w26) -> ()
      n14 = case shown="1" w21 {
        tunnel: [T20."Disabled and Grayed Out" ("禁用") T20."Enabled" ("禁用")] -> w27
        frame 0, Default {
        }
        frame 1 {
        }
      }
      n15 = local write "Channel"(w20) -> ()
      n16 = case shown="1" w21 {
        tunnel: w25 -> [w39 w41]
        tunnel: w24 -> [w38 _]
        tunnel: w23 -> [_ w40]
        tunnel: w22 -> [_ _]
        frame 0, Default {
          n17 = call "TSCAN_Table.vi"("Buffer"=w38, "MCListbox reference handle"=w39) -> ()  [unwired: 10 in]
        }
        frame 1 {
          n18 = call "TSCANfd_Table.vi"("Messages"=w40, "MCListbox reference handle"=w41) -> ()  [unwired: 10 in]
        }
      }
      n19 = property on="BRS" class="Enum (严格)"("DisabledEnum"=w27) -> ()  [unwired: 2 in, 2 out]
      n20 = property on="FD Frame" class="Ring (严格)"("DisabledEnum"=w27) -> ()  [unwired: 2 in, 2 out]
    }
  }
  n21 = Unbundle By Name(w3) -> ("Communication message"=w1:T18)
  n22 = Create User Event(user event datatype=w9) -> (user event=w6:refnum<user-event>)  [unwired: 1 in, 1 out]
  n23 = register-events(w6) -> (reference out=w8:refnum<event-registration>)  [unwired: 2 in, 1 out]
  n24 = Obtain Queue(name (unnamed)="Sender", element data type=T18 {"Sender"="", "receiver"="", "message"="", "data"=variant} ("Communication message")) -> (queue out=w19:refnum<queue>, error out=w12:errorcluster)  [unwired: 3 in, 1 out]
  n25 = Bundle By Name(cluster=w3, "Communication message.Sender"="Sender") -> (w11:T2)
  n26 = while {
    tunnel: w19 -> [w51]
    tunnel: w12 -> [w49]
    tunnel: "Sender" -> [w45]
    tunnel: w8 -> [w44]
    stop <- w52 stop-if-true
    n27 = event shown="[2] \"Add\": 值改变" {
      selector: w44 -> [_ _ _ _ _ _ _ _]
      dyn-events: _ -> [_ _ _ _ _ _ _ _]
      timeout: _ -> [_ _ _ _ _ _ _ _]
      tunnel: [_ _ _ _ _ w92 w99 TRUE ("放弃？")] -> w52
      tunnel: w51 -> [w62 w77 w81 w85 w91 w95 w98 w102]
      tunnel: [w62 w77 w81 w85 w91 w95 w96 w100] -> w50
      tunnel: [T18 {"Sender"="", "receiver"="", "message"="", "data"=variant} ("Communication message") w73 w78 w82 w88 _ _ _] -> w47
      tunnel: [w61 _ _ _ _ _ _ _] -> w48
      tunnel: w49 -> [w61 _ _ _ _ _ _ _]
      tunnel: w45 -> [_ _ _ _ _ _ _ _]
      event Timeout {
        n28 = event-data() -> ()  [unwired: 1 in, 3 out]
      }
      event "SendData", "Data Length", "ID", "Frame Format", "Frame Type", "FD Frame", "BRS", "Channel": Value Change {
        n29 = event-data() -> ()  [unwired: 1 in, 6 out]
        n30 = Bundle By Name(cluster=T2 {"Communication message"={"Sender"="", "receiver"="", "message"="", "data"=variant}, "Data"={"Config_parameter"={"Bus_Type"=0, "Channel"=0, "Channels used"=0, "DLL_PATH"=path "", "Read message type"=0, "REC_Channel"=0}, "Send_parameter"={"SendData"=[], "Data Length"=0, "ID"=0, "Frame Format"=0, "Frame Type"=0, "BRS"=enum."Close", "FD Frame"=0, "async&sync"=enum."async", "Timeout"=0}, "DBC_Ctr"={"DBC Path"=path "", "DBC loading channel"=0, "DatabaseId"=0, "DBMessages"=[], "DBSignals"=[]}, "CAN_Config_Array"=[], "CANFD_Config_Array"=[], "CAN_Config_Regs_Array"=[], "CANFD_Config_Regs_Array"=[], "Blf_Log"={"Blf_Log_PATH"=path ""}, "UDS"={"UDS Control"={"UDS Channel Index"=0, "Request ID"=1992, "Response ID"=2015, "Request ID (Func)"=1, "Session Mode"=1, "Reset Mode"=255, "DTC Mask"=0, "GropOfDTC"=0, "Seed Level"=2, "Seed"=[], "Key Level"=0, "Key"=[], "Read Identifier"=0, "UDS Read Data"=[], "ASCII Data"="", "Write Identifier"=0, "UDS Wrtie Data"=[], "IO Control Identifier"=1, "UDS IOControl Data"=[], "IO Control Mode"=0, "UDS IOControl Read Data"=[], "Routine Control Identifier"=0, "UDS RoutineControl Data"=[], "UDS RoutineControl Read Data"=[], "Routine Control Mode"=1, "SupportFDCAN"=TRUE, "time config"={"p2_timeout"=0, "p2_extended"=0, "s3_servertime"=0, "s3_clienttime"=0}, "ServiceLayer"={"FilledByte"=0, "STMin"=10, "BlockSize"=10, "FCDelay"=10, "MaxLength"=4095}, "Request"=[], "Respond"=[]}, "DiagModuleIndex"=1984}}, "CAN_Buffer"=[], "CANFD_Buffer"=[], "error in"={"status"=FALSE, "code"=0, "source"=""}, "CAN_Period_Datas"=[], "CANFD_period_Datas"=[], "CAN_Filtering_Datas"=[], "CANFD_Filtering_Datas"=[], "AsynCall?"=FALSE} ("Data"), "Data.Config_parameter.Channel"="Channel", "Data.Send_parameter.SendData"="SendData", "Data.Send_parameter.Data Length"="Data Length", "Data.Send_parameter.ID"="ID", "Data.Send_parameter.Frame Format"="Frame Format", "Data.Send_parameter.Frame Type"="Frame Type", "Data.Send_parameter.BRS"="BRS", "Data.Send_parameter.FD Frame"="FD Frame") -> (w64:T2)
        n31 = To Variant(anything=w64) -> (Variant=w75:variant)
        n32 = Bundle By Name(cluster=T18 {"Sender"="", "receiver"="", "message"="", "data"=variant} ("Communication message"), "message"="Config update", "data"=w75) -> (w73:T18)
      }
      event "Add": Value Change {
        n33 = event-data() -> ()  [unwired: 1 in, 6 out]
        n34 = Bundle By Name(cluster=T18 {"Sender"="", "receiver"="", "message"="", "data"=variant} ("Communication message"), "message"="Add") -> (w78:T18)
      }
      event "Remove": Value Change {
        n35 = event-data() -> ()  [unwired: 1 in, 6 out]
        n36 = Bundle By Name(cluster=T18 {"Sender"="", "receiver"="", "message"="", "data"=variant} ("Communication message"), "message"="Remove") -> (w82:T18)
      }
      event "Data_Display": Value Change {
        n37 = event-data() -> ("NewVal"=w86:i32)  [unwired: 1 in, 5 out]
        n38 = To Variant(anything=w86) -> (Variant=w87:variant)
        n39 = Bundle By Name(cluster=T18 {"Sender"="", "receiver"="", "message"="", "data"=variant} ("Communication message"), "message"="Data_Display", "data"=w87) -> (w88:T18)
      }
      event User Event {
        n40 = event-data() -> ("Message"=w94:string)  [unwired: 1 in]
        n41 = Equal?(x=w94, y="Quit") -> (x = y?=w92:bool)
      }
      event Panel Close? {
        w99 = TRUE ("放弃？")
        n42 = event-data() -> ()  [unwired: 1 in, 4 out]
        n43 = Enqueue Element(queue=w98, element=T18 {"Sender"="", "receiver"="", "message"="Quit", "data"=variant} ("Communication message")) -> (queue out=w96:refnum<queue>)  [unwired: 2 in, 2 out]
        n44 = event-data("Discard?"=w99) -> ()  [unwired: 1 in, 1 out]
      }
      event "STOP": Value Change {
        n45 = event-data() -> ()  [unwired: 1 in, 6 out]
        n46 = Enqueue Element(queue=w102, element=T18 {"Sender"="", "receiver"="", "message"="Quit", "data"=variant} ("Communication message")) -> (queue out=w100:refnum<queue>)  [unwired: 2 in, 2 out]
      }
    }
    n47 = Unbundle By Name(w47) -> ("message"=w46:string)
    n48 = case shown="\"default\", 默认" w46 {
      tunnel: w50 -> [w57 w59]
      tunnel: w48 -> [w56 w58]
      tunnel: w47 -> [w55 _]
      tunnel: [w54 w59] -> _
      tunnel: [w53 w58] -> _
      frame "default", Default {
        n49 = Enqueue Element(queue=w57, element=w55, error in (no error)=w56) -> (queue out=w54:refnum<queue>, error out=w53:errorcluster)  [unwired: 1 in, 1 out]
      }
      frame "" {
      }
    }
  }
  n50 = while {
    tunnel: w19 -> [w123]
    tunnel: w12 -> [w122]
    tunnel: [w114] -> w18
    tunnel: [w113] -> w17
    shift-right: [w108] -> w5
    shift-left: w11 -> [w109]
    tunnel: w8 -> [w107]
    tunnel: w7 -> [_]
    tunnel: w6 -> [w106]
    shift-right: [w105] -> _
    shift-left: -1 ("新值") -> [w104]
    stop <- w112 stop-if-true
    n51 = Dequeue Element(queue=w123, error in (no error)=w122) -> (queue out=w119:refnum<queue>, element=w121:T18, error out=w118:errorcluster)  [unwired: 1 in, 1 out]
    n52 = Unbundle By Name(w121) -> ("message"=w120:string, "data"=w115:variant)
    n53 = case shown="\"Add\"" w120 {
      tunnel: [w138 w142 w145 w162 w206 w231 w242] -> w117
      tunnel: w119 -> [w138 w142 w145 w162 w206 w231 w241]
      tunnel: w118 -> [w137 w141 w146 w163 w205 w230 w239]
      tunnel: [w137 w141 w146 w163 w205 w230 w240] -> w116
      tunnel: w115 -> [_ _ w157 _ _ w228 _]
      tunnel: [_ _ _ _ _ _ TRUE] -> w112
      tunnel: [w135 _ _ _ _ _ _] -> w111
      tunnel: [w132 w140 w154 w159 w198 w229 w238] -> w108
      tunnel: w109 -> [w132 w140 w156 w164 w202 w229 w238]
      tunnel: w107 -> [_ _ _ _ _ _ w233]
      tunnel: w106 -> [_ _ _ _ _ _ w234]
      tunnel: [w131 w139 w144 w160 w201 w226 w232] -> w105
      tunnel: w104 -> [w131 w139 w144 w160 w201 _ w232]
      frame "eee", Default {
        w133 = ""
        n54 = Bundle By Name(cluster=T18 {"Sender"="", "receiver"="", "message"="", "data"=variant} ("Communication message"), "Sender"=w133, "receiver"=w133, "message"=w133, "data"=variant) -> (w135:T18)
      }
      frame "Init" {
      }
      frame "Config update" {
        n55 = Variant To Data(type=w156, Variant=w157) -> (data=w155:T2)  [unwired: 1 in, 1 out]
        n56 = Unbundle By Name(w155) -> ("Data.Send_parameter.SendData"=w153:u8[], "Data.Send_parameter.Data Length"=w152:i32, "Data.Send_parameter.ID"=w151:i32, "Data.Send_parameter.Frame Format"=w150:u8, "Data.Send_parameter.Frame Type"=w149:u8, "Data.Send_parameter.BRS"=w148:enum16{"Close", "Open"}, "Data.Send_parameter.FD Frame"=w147:u8, "Data.Config_parameter.Channel"=w143:i32)
        n57 = Bundle By Name(cluster=w156, "Data.Send_parameter.SendData"=w153, "Data.Send_parameter.Data Length"=w152, "Data.Send_parameter.ID"=w151, "Data.Send_parameter.Frame Format"=w150, "Data.Send_parameter.Frame Type"=w149, "Data.Send_parameter.BRS"=w148, "Data.Send_parameter.FD Frame"=w147, "Data.Config_parameter.Channel"=w143) -> (w154:T2)
      }
      frame "Add" {
        n58 = control-ref of="Data_Display"() -> (w161:refnum<vi>)
        n59 = Unbundle By Name(w164) -> ("Data.Config_parameter.DLL_PATH"=w166:path, "Data.Config_parameter.Bus_Type"=w167:u16)
        n60 = case shown="1" w167 {
          tunnel: w166 -> [w181 w197]
          tunnel: "APeriodMS" -> [w168 w182]
          tunnel: w164 -> [w171 w187]
          tunnel: w161 -> [w172 w185]
          tunnel: [w169 w186] -> w159
          frame 0, Default {
            n61 = Unbundle By Name(w171) -> ("Data.Config_parameter.Channel"=w180:i32, "Data.Send_parameter.ID"=w179:i32, "Data.Send_parameter.Frame Format"=w178:u8, "Data.Send_parameter.Frame Type"=w177:u8, "Data.Send_parameter.Data Length"=w176:i32, "Data.Send_parameter.SendData"=w174:u8[])
            n62 = Array To Cluster(array=w174) -> (cluster=w175:T24)
            n63 = Bundle By Name(cluster=T22 {"AIdxchn"=0, "AId"=0, "AIsStd"=0, "AIsData"=0, "ADLC"=0, "ADataArray"={"Data0"=0, "Data1"=0, "Data2"=0, "Data3"=0, "Data4"=0, "Data5"=0, "Data6"=0, "Data7"=0}} ("TCAN"), "AIdxchn"=w180, "AId"=w179, "AIsStd"=w178, "AIsData"=w177, "ADLC"=w176, "ADataArray"=w175) -> (w170:T22)
            n64 = call "tsapp_add_cyclic_msg_can.vi"("APeriodMS"=w168, "TCAN"=w170, "path"=w181) -> ()  [unwired: 6 in, 3 out]
            n65 = call "TSCAN_Periodic_Sending_CAN_Table.vi"("FTimeUS"=w168, "TCAN"=w170, "多列列表框输入"=w172, "Data输入"=w171) -> ("Data输出"=w169:T2)  [unwired: 7 in]
          }
          frame 1 {
            n66 = Unbundle By Name(w187) -> ("Data.Config_parameter.Channel"=w195:i32, "Data.Send_parameter.ID"=w194:i32, "Data.Send_parameter.Frame Format"=w193:u8, "Data.Send_parameter.Frame Type"=w183:u8, "Data.Send_parameter.Data Length"=w192:i32, "Data.Send_parameter.FD Frame"=w191:u8, "Data.Send_parameter.BRS"=w189:enum16{"Close", "Open"}, "Data.Send_parameter.SendData"=w188:u8[])
            n67 = Array To Cluster(array=w188) -> (cluster=w190:T25)
            n68 = Bundle By Name(cluster=T23 {"AIdxchn"=0, "AId"=0, "AIsStd"=0, "BRS"=enum."Close", "AIsData"=0, "ADLC"=0, "AIsFD"=enum."Classic CAN Message", "FDatas"={"Initialize array[0]"=0, "Initialize array[1]"=0, "Initialize array[2]"=0, "Initialize array[3]"=0, "Initialize array[4]"=0, "Initialize array[5]"=0, "Initialize array[6]"=0, "Initialize array[7]"=0, "Initialize array[8]"=0, "Initialize array[9]"=0, "Initialize array[10]"=0, "Initialize array[11]"=0, "Initialize array[12]"=0, "Initialize array[13]"=0, "Initialize array[14]"=0, "Initialize array[15]"=0, "Initialize array[16]"=0, "Initialize array[17]"=0, "Initialize array[18]"=0, "Initialize array[19]"=0, "Initialize array[20]"=0, "Initialize array[21]"=0, "Initialize array[22]"=0, "Initialize array[23]"=0, "Initialize array[24]"=0, "Initialize array[25]"=0, "Initialize array[26]"=0, "Initialize array[27]"=0, "Initialize array[28]"=0, "Initialize array[29]"=0, "Initialize array[30]"=0, "Initialize array[31]"=0, "Initialize array[32]"=0, "Initialize array[33]"=0, "Initialize array[34]"=0, "Initialize array[35]"=0, "Initialize array[36]"=0, "Initialize array[37]"=0, "Initialize array[38]"=0, "Initialize array[39]"=0, "Initialize array[40]"=0, "Initialize array[41]"=0, "Initialize array[42]"=0, "Initialize array[43]"=0, "Initialize array[44]"=0, "Initialize array[45]"=0, "Initialize array[46]"=0, "Initialize array[47]"=0, "Initialize array[48]"=0, "Initialize array[49]"=0, "Initialize array[50]"=0, "Initialize array[51]"=0, "Initialize array[52]"=0, "Initialize array[53]"=0, "Initialize array[54]"=0, "Initialize array[55]"=0, "Initialize array[56]"=0, "Initialize array[57]"=0, "Initialize array[58]"=0, "Initialize array[59]"=0, "Initialize array[60]"=0, "Initialize array[61]"=0, "Initialize array[62]"=0, "Initialize array[63]"=0}} ("TCANFD"), "AIdxchn"=w195, "AId"=w194, "AIsStd"=w193, "AIsData"=w183, "ADLC"=w192, "AIsFD"=w191, "FDatas"=w190, "BRS"=w189) -> (w184:T23)
            n69 = call "tsapp_add_cyclic_msg_canfd.vi"("APeriodMS"=w182, "TCANFD"=w184, "Path"=w197) -> ()  [unwired: 6 in, 3 out]
            n70 = call "TSCAN_Periodic_Sending_CANFD_Table.vi"("FTimeUS"=w182, "TCANFD"=w184, "多列列表框输入"=w185, "Data in"=w187) -> ("Data输出"=w186:T2)  [unwired: 7 in]
          }
        }
        n71 = Unbundle By Name(w159) -> ("CAN_Period_Datas"=→"CAN_Period_Datas":T1)
      }
      frame "Remove" {
        n72 = Unbundle By Name(w202) -> ("Data.Config_parameter.DLL_PATH"=w203:path, "Data.Config_parameter.Bus_Type"=w204:u16)
        n73 = control-ref of="Data_Display"() -> (w200:refnum<vi>)
        n74 = case shown="0, 默认" w204 {
          tunnel: w203 -> [w214 w220]
          tunnel: [w210 w217] -> w198
          tunnel: w202 -> [w211 w218]
          tunnel: w201 -> [w212 w219]
          tunnel: w200 -> [w209 w221]
          frame 0, Default {
            n75 = Unbundle By Name(w211) -> ("CAN_Period_Datas"=w213:T1)
            n76 = call "TSCAN_Periodic_Sending_DeleCAN_Table.vi"("Data"=w211, "value"=w212, "DLL_PATH"=w214) -> ()  [unwired: 8 in, 1 out]
            n77 = Delete From Array(array=w213, index=w212) -> (array with subset deleted=w208:T1)  [unwired: 1 in, 1 out]
            n78 = Bundle By Name(cluster=w211, "CAN_Period_Datas"=w208) -> (w210:T2)
            n79 = call "TSCAN_Table.vi"("ms?"=TRUE, "Buffer"=w208, "MCListbox reference handle"=w209) -> ()  [unwired: 9 in]
          }
          frame 1 {
            n80 = Unbundle By Name(w218) -> ("CANFD_period_Datas"=w222:T21)
            n81 = disable-structure shown="启用" {
              disable-tunnel: w220 -> [w225 _]
              disable-tunnel: w219 -> [w224 _]
              disable-tunnel: w218 -> [w223 _]
              frame Enabled {
                n82 = call "TSCAN_Periodic_Sending_DeleCANFD_Table.vi"("Data"=w223, "value"=w224, "DLL_PATH"=w225) -> ()  [unwired: 8 in, 1 out]
              }
              frame Disabled {
              }
            }
            n83 = Delete From Array(array=w222, index=w219) -> (array with subset deleted=w216:T21)  [unwired: 1 in, 1 out]
            n84 = Bundle By Name(cluster=w218, "CANFD_period_Datas"=w216) -> (w217:T2)
            n85 = call "TSCANfd_Table.vi"("ms?"=TRUE, "Messages"=w216, "MCListbox reference handle"=w221) -> ()  [unwired: 9 in]
          }
        }
        n86 = Unbundle By Name(w198) -> ("CAN_Period_Datas"=w199:T1)
        n87 = local write "CAN_Period_Datas"(w199) -> ()
      }
      frame "Data_Display" {
        n88 = Variant To Data(type=0 ("新值"), Variant=w228) -> (data=w226:i32)  [unwired: 1 in, 1 out]
      }
      frame "Quit" {
        n89 = Generate User Event(user event=w234, event data cluster="Quit" ("y")) -> (user event out=w236:refnum<user-event>, error out=w235:errorcluster)  [unwired: 2 in]
        n90 = register-events(reference=w233, error in=w235, w236) -> ()  [unwired: 2 out]
        n91 = Flush Queue(queue=w241, error in (no error)=w239) -> (queue out=w242:refnum<queue>, error out=w240:errorcluster)  [unwired: 1 out]
      }
    }
    n92 = Unbundle By Name(w111) -> ("message"=w110:string)
    n93 = case shown="\"default\", 默认" w110 {
      tunnel: w117 -> [w128 w130]
      tunnel: w116 -> [w127 w129]
      tunnel: w111 -> [w126 _]
      tunnel: [w125 w130] -> w114
      tunnel: [w124 w129] -> w113
      frame "default", Default {
        n94 = Enqueue Element(queue=w128, element=w126, error in (no error)=w127) -> (queue out=w125:refnum<queue>, error out=w124:errorcluster)  [unwired: 1 in, 1 out]
      }
      frame "" {
      }
    }
  }
  n95 = Release Queue(queue=w18, error in (no error)=w17) -> (error out=w16:errorcluster)  [unwired: 1 in, 2 out]
  n96 = Bundle By Name(cluster=w5, "Communication message"=w1) -> (→"Data 2":T2)
  n97 = property class="App"(error in=w16) -> (error out=w15:errorcluster, "App.Kind"=w14:T26)  [unwired: 1 in, 1 out]
  n98 = case shown="\"Run Time System\"" w14 {
    tunnel: w15 -> [_ _ w244 _ _ _ _]
    frame "invalid app kind", Default {
    }
    frame "Development System" {
    }
    frame "Run Time System" {
      n99 = invoke class="VI" method="FP.Close"(error in=w244) -> ()  [unwired: 2 in, 3 out]
    }
    frame "Student Edition" {
    }
    frame "Embedded LabVIEW" {
    }
    frame "Evaluation" {
    }
    frame "Custom" {
    }
  }
